vi "S7_Close.vi"(8 "error in":errorcluster, 11 "TCP Connection Ref":refnum<k5>) -> (0 "error out":errorcluster)   [LabVIEW 2018]
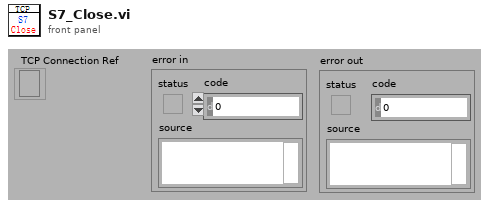
[diagram p1: front panel]
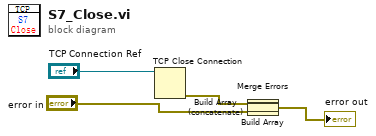
[diagram p0: block diagram]
diagram:
  n1 = TCP Close Connection(connection ID="TCP Connection Ref") -> (error out=w5:errorcluster)  [unwired: 1 in, 2 out]
  n2 = Build Array(w5, "error in") -> (w2:errorcluster[])
  n3 = Build Array (concatenate)(w2) -> (w1:errorcluster[])
  n4 = Merge Errors(w1) -> (→"error out":errorcluster)
